vi "3_WF_Anomaly_Detection(Accuracy_Evaluation).vi"() -> ()   [LabVIEW 2020]
uses:
  <vilib>/Ngene/Deep Learning Toolkit/Toolkit/NN_Data/subVIs/Dataset/NN_Variant_to_DVR/2D/NN_Data_Variant_to_DVR(2D_SGL).vi
  <vilib>/Ngene/Deep Learning Toolkit/Toolkit/NN_Network/subVIs/NN_Predict/NN_Predict(In1D_Out1D).vi
  <vilib>/Ngene/Deep Learning Toolkit/Toolkit/NN_Data/subVIs/Get_Data_Vals/2D/NN_Data_Get_ValByRef(2D_SGL).vi
  <vilib>/Ngene/Deep Learning Toolkit/Toolkit/Deep_Learning_Toolkit_by_Ngene.lvlib
  <vilib>/Analysis/NI_AALPro.lvlib
panel:
  out "Error Rate":sgl
  in  "Labels":string[](array[string])=["Normal", "Abnormal"]
  in  "Optimal Threshold":sgl=0.2
  out "Anomaly Score Distribution":T1(graph)=[{"X Values"=array[700 elements], "Histogram: h(x)"=[0, 0, 0, 0, 0, 0, 0, 0, 0, 0, 0, 0, 0, 0, 0, 0, 0, 0, 0, 0, 0, 0, 0, 0, 0, 0, 0, 0, 0, 0, 0, 0, 0, 0, 0, 1, 0, 1, 2, 2, 7, 7, 7, 4, 17, 6, 12, 11, 9, 10, 15, 15, 11, 18, 18, 18, 13, 13, 16, 11, 14, 20, 11, 9, 16, 11, 16, 10, 11, 9, 8, 15, 6, 8, 4, 10, 3, 4, 1, 6, 3, 6, 3, 10, 6, 5, 3, 1, 5, 2, 1, 2, 1, 4, 2, 2, 1, 1, 0, 1, 0, 0, 1, 0, 0, 0, 1, 1, 0, 0, 0, 0, 0, 0, 0, 0, 1, 0, 0, 0, 0, 0, 0, 1, 0, 0, 0, 0, 0, 0, 0, 0, 0, 0, 0, 0, 0, 0, 0, 0, 0, 0, 0, 0, 0, 0, 0, 0, 0, 0, 0, 0, 0, 0, 0, 0, 0, 0, 0, 0, 0, 0, 0, 0, 0, 0, 0, 0, 0, 0, 0, 0, 0, 0, 0, 0, 0, 0, 0, 0, 0, 0, 0, 0, 0, 0, 0, 0, 0, 0, 0, 0, 0, 0, 0, 0, 0, 0, 0, 0, 0, 0, 0, 0, 0, 0, 0, 0, 0, 0, 0, 0, 0, 0, 0, 0, 0, 0, 0, 0, 0, 0, 0, 0, 0, 0, 0, 0, 0, 0, 0, 0, 0, 0, 0, 0, 0, 0, 0, 0, 0, 0, 0, 0, 0, 0, 0, 0, 0, 0, 0, 0, 0, 0, 0, 0, 0, 0, 0, 0, 0, 0, 0, 0, 0, 0, 0, 0, 0, 0, 0, 0, 0, 0, 0, 0, 0, 0, 0, 0, 0, 0, 0, 0, 0, 0, 0, 0, 0, 0, 0, 0, 0, 0, 0, 0, 0, 0, 0, 0, 0, 0, 0, 0, 0, 0, 0, 0, 0, 0, 0, 0, 0, 0, 0, 0, 0, 0, 0, 0, 0, 0, 0, 0, 0, 0, 0, 0, 0, 0, 0, 0, 0, 0, 0, 0, 0, 0, 0, 0, 0, 0, 0, 0, 0, 0, 0, 0, 0, 0, 0, 0, 0, 0, 0, 0, 0, 0, 0, 0, 0, 0, 0, 0, 0, 0, 0, 0, 0, 0, 0, 0, 0, 0, 0, 0, 0, 0, 0, 0, 0, 0, 0, 0, 0, 0, 0, 0, 0, 0, 0, 0, 0, 0, 0, 0, 0, 0, 0, 0, 0, 0, 0, 0, 0, 0, 0, 0, 0, 0, 0, 0, 0, 0, 0, 0, 0, 0, 0, 0, 0, 0, 0, 0, 0, 0, 0, 0, 0, 0, 0, 0, 0, 0, 0, 0, 0, 0, 0, 0, 0, 0, 0, 0, 0, 0, 0, 0, 0, 0, 0, 0, 0, 0, 0, 0, 0, 0, 0, 0, 0, 0, 0, 0, 0, 0, 0, 0, 0, 0, 0, 0, 0, 0, 0, 0, 0, 0, 0, 0, 0, 0, 0, 0, 0, 0, 0, 0, 0, 0, 0, 0, 0, 0, 0, 0, 0, 0, 0, 0, 0, 0, 0, 0, 0, 0, 0, 0, 0, 0, 0, 0, 0, 0, 0, 0, 0, 0, 0, 0, 0, 0, 0, 0, 0, 0, 0, 0, 0, 0, 0, 0, 0, 0, 0, 0, 0, 0, 0, 0, 0, 0, 0, 0, 0, 0, 0, 0, 0, 0, 0, 0, 0, 0, 0, 0, 0, 0, 0, 0, 0, 0, 0, 0, 0, 0, 0, 0, 0, 0, 0, 0, 0, 0, 0, 0, 0, 0, 0, 0, 0, 0, 0, 0, 0, 0, 0, 0, 0, 0, 0, 0, 0, 0, 0, 0, 0, 0, 0, 0, 0, 0, 0, 0, 0, 0, 0, 0, 0, 0, 0, 0, 0, 0, 0, 0, 0, 0, 0, 0, 0, 0, 0, 0, 0, 0, 0, 0, 0, 0, 0, 0, 0, 0, 0, 0, 0, 0, 0, 0, 0, 0, 0, 0, 0, 0, 0, 0, 0, 0, 0, 0, 0, 0, 0, 0, 0, 0, 0, 0, 0, 0, 0, 0, 0, 0, 0, 0, 0, 0, 0, 0, 0, 0, 0, 0, 0, 0, 0, 0, 0, 0, 0, 0, 0, 0, 0, 0, 0, 0, 0, 0, 0, 0, 0, 0, 0, 0, 0, 0]}, {"X Values"=array[700 elements], "Histogram: h(x)"=[0, 0, 0, 0, 0, 0, 0, 0, 0, 0, 0, 0, 0, 0, 0, 0, 0, 0, 0, 0, 0, 0, 0, 0, 0, 0, 0, 0, 0, 0, 0, 0, 0, 0, 0, 0, 0, 0, 0, 0, 0, 0, 0, 0, 0, 0, 0, 0, 0, 0, 0, 0, 0, 0, 0, 0, 0, 0, 0, 0, 0, 0, 0, 0, 0, 0, 0, 0, 0, 0, 0, 0, 0, 0, 0, 0, 0, 0, 0, 0, 0, 0, 0, 0, 0, 0, 0, 0, 0, 0, 0, 0, 0, 0, 0, 0, 0, 0, 0, 0, 0, 0, 0, 0, 0, 0, 0, 0, 0, 0, 0, 0, 0, 0, 0, 0, 0, 0, 0, 0, 0, 0, 0, 0, 0, 0, 0, 0, 0, 0, 0, 0, 0, 0, 0, 0, 0, 0, 0, 0, 0, 0, 0, 0, 0, 0, 0, 0, 0, 0, 0, 0, 0, 0, 0, 0, 0, 0, 0, 0, 0, 0, 0, 0, 0, 0, 0, 0, 0, 1, 0, 0, 0, 0, 0, 2, 0, 0, 0, 0, 0, 0, 0, 0, 1, 1, 2, 1, 2, 0, 2, 0, 1, 0, 0, 0, 1, 1, 1, 1, 2, 3, 2, 0, 1, 0, 2, 3, 1, 2, 0, 4, 4, 1, 0, 1, 1, 0, 0, 0, 1, 0, 4, 3, 2, 5, 2, 2, 1, 1, 2, 1, 4, 3, 2, 1, 2, 5, 0, 4, 1, 1, 3, 2, 2, 2, 1, 2, 6, 2, 1, 0, 0, 2, 1, 3, 2, 3, 6, 1, 4, 5, 0, 1, 1, 4, 3, 2, 5, 2, 2, 0, 1, 0, 2, 0, 2, 4, 0, 2, 0, 2, 0, 4, 1, 0, 1, 1, 0, 1, 1, 3, 3, 1, 0, 0, 3, 1, 1, 0, 1, 1, 1, 4, 2, 2, 3, 0, 1, 1, 3, 1, 1, 0, 0, 0, 2, 0, 1, 3, 1, 0, 1, 1, 1, 0, 1, 0, 1, 1, 0, 0, 0, 0, 1, 2, 1, 0, 1, 0, 0, 0, 0, 0, 0, 0, 3, 2, 0, 0, 0, 1, 0, 0, 0, 2, 0, 0, 1, 0, 1, 2, 2, 4, 2, 1, 2, 3, 1, 1, 3, 0, 1, 3, 1, 2, 0, 1, 0, 1, 0, 2, 1, 1, 1, 2, 1, 0, 2, 0, 1, 1, 2, 4, 4, 2, 2, 0, 1, 2, 1, 1, 1, 1, 1, 1, 1, 1, 2, 1, 1, 1, 1, 5, 3, 1, 1, 1, 4, 2, 3, 1, 0, 0, 1, 0, 0, 0, 1, 5, 2, 1, 2, 1, 1, 3, 0, 3, 2, 2, 0, 1, 1, 2, 1, 0, 2, 1, 2, 0, 1, 0, 1, 2, 0, 1, 0, 0, 2, 0, 0, 0, 2, 1, 2, 1, 2, 1, 1, 1, 1, 0, 1, 1, 0, 1, 1, 0, 1, 1, 0, 0, 0, 0, 0, 1, 0, 0, 0, 1, 0, 0, 0, 0, 0, 0, 0, 0, 0, 0, 0, 1, 0, 0, 0, 0, 0, 0, 0, 0, 0, 1, 0, 0, 0, 0, 0, 0, 0, 0, 0, 0, 0, 0, 0, 0, 0, 0, 0, 0, 0, 0, 0, 0, 0, 0, 1, 0, 0, 0, 0, 0, 0, 0, 0, 0, 0, 0, 0, 0, 0, 0, 0, 0, 0, 0, 0, 0, 0, 0, 0, 0, 0, 0, 0, 0, 0, 1, 1, 0, 0, 0, 0, 0, 1, 1, 1, 0, 0, 0, 0, 0, 0, 1, 0, 0, 3, 0, 1, 0, 0, 0, 0, 2, 2, 0, 4, 0, 3, 3, 1, 0, 1, 4, 4, 1, 3, 1, 0, 2, 1, 2, 1, 3, 1, 1, 0, 1, 0, 5, 2, 4, 4, 2, 1, 1, 0, 1, 1, 2, 1, 2, 3, 2, 1, 1, 1, 3, 0, 0, 1, 4, 1, 0, 0, 2, 0, 0, 2, 0, 0, 0, 0, 0, 0, 1, 0, 0, 1, 0, 0, 0, 0, 0, 0, 0, 0, 0, 0, 0, 0, 0, 0, 0, 0, 0, 0, 0, 0, 0, 0, 0, 0, 0, 0, 0, 0, 0, 0, 0, 0, 0, 0, 0, 0, 0, 0, 0, 0, 0]}]
  in  "Test (Normal Samples) Dataset Folder path":path=path "D:/working/Anomaly Detection/Test/Normal"
  out "Confusion Matrix (Table)":string[][](table)=[["500", "0", "1.0000"], ["0", "500", "1.0000"], ["1.0000", "1.0000", ""]]
  in  "Test (Abnormal Samples) Dataset Folder path":path=path "D:/working/Anomaly Detection/Test/Abnormal"
  in  "Weights File Path":path=path "D:/Ngene/GitHub/deepltk_examples/2_Waveform_Processing/24_Waveform_Anomaly_Detection/working/Anomaly_Detection/Anomaly_Detection_weights_25_06_11__13_26_24.bin"
  in  "CFG file path":path=path "D:/Ngene/GitHub/deepltk_examples/2_Waveform_Processing/24_Waveform_Anomaly_Detection/working/Anomaly_Detection/Anomaly_Detection_net_cfg_25_06_11__13_26_24.cfg"
  # "Overview: This VI is designed to calculate the optimal anomaly threshold on the generated synthetic dataset.\nRequirements: Deep Learning Toolkit for LabVIEW - https://www.ngene.co/deep-learning-toolkit-for-labview\nInstructions:\n1. Provide \"Network Configuration File Path\" and \"Weight File Path\" generated from \"1_WF_Anomaly_Detection(Training).vi\".\n2. Provide Train and Test dataset paths.\n3. Run the VI.\n4.Observe the Range of optimal threshold values.\n5. Choose a value from the range of optimal threshold calculated after the VI stops, and use it as a anomaly detetcion threshold in \"3_WF_Anomaly_Detection(Threshold_Evaluation).vi\" \n6. Open \"3_WF_Anomaly_Detection(Inference).vi\"  to deploy the trained network for inference on manually generated samples."
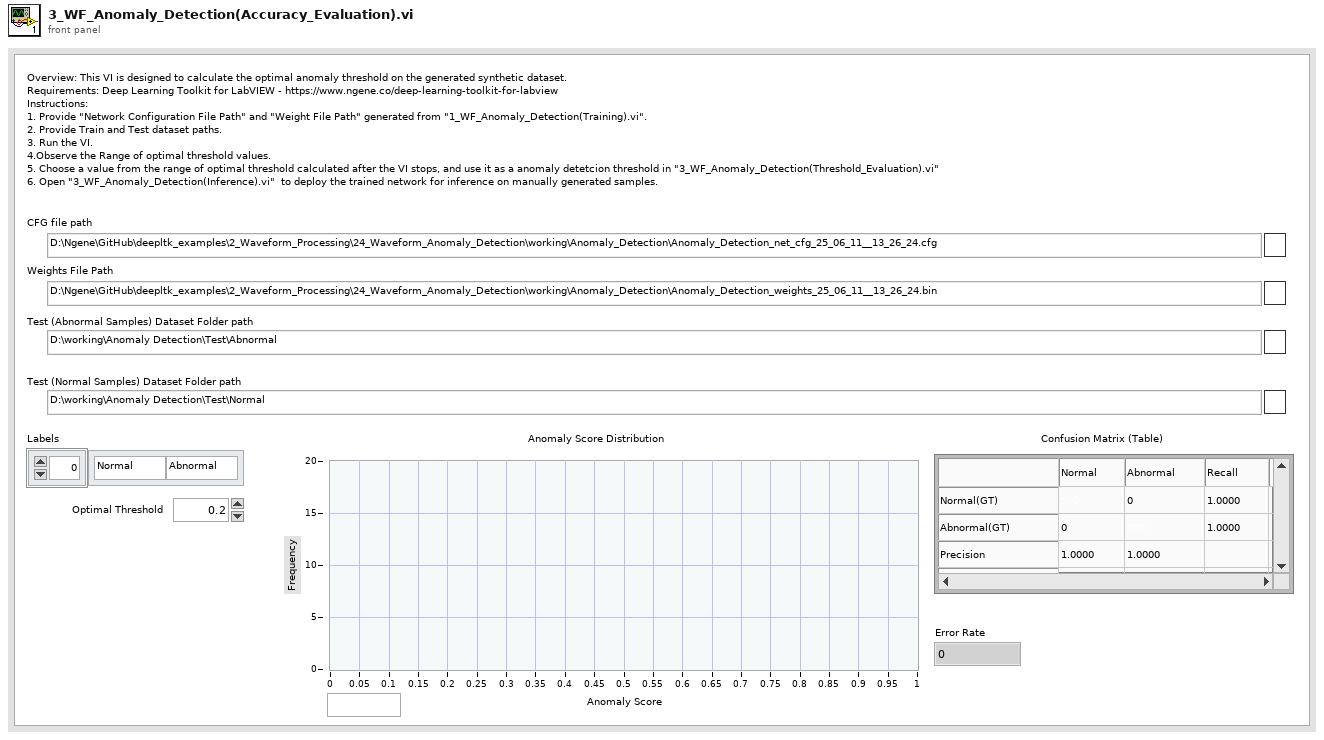
[diagram p1: front panel]
types:
  T1 = cluster{"X Values":dbl[], "Histogram: h(x)":i32[]}[]
  T2 = typedef "Deep_Learning_Toolkit_by_Ngene.lvlib/NN_Config_Params.ctl" = cluster{"Name":string, "mBatch":i32, "NN_Train_Params":T3, "LR_Decay_Policy":T6, "Labels":string[], "Loss":T8}
  T3 = typedef "Deep_Learning_Toolkit_by_Ngene.lvlib/NN_Train_Params.ctl" = cluster{"Optimizer":T4, "Beta_1":sgl, "Beta_2":sgl, "Weight Decay(L1)":sgl, "Weight Decay(L2)":sgl, "Data_Sampling":T5}
  T4 = typedef "Deep_Learning_Toolkit_by_Ngene.lvlib/NN_Train_Optimizer.ctl" = enum16{"SGD", "Adam", "Adagrad", "Adadelta", "RMSProp", "Nesterov"}
  T5 = typedef "Deep_Learning_Toolkit_by_Ngene.lvlib/NN_Train_Data_Sampling.ctl" = enum16{"Random", "Sequential"}
  T6 = typedef "Deep_Learning_Toolkit_by_Ngene.lvlib/NN_LR_Policy_Cfg.ctl" = cluster{"Policy_Type":T7, "LR0":dbl, "k":sgl, "WarmUp_Policy":enum16{"Step", "Ramp"}, "WarmUp_Iter":i32, "WarmUp_Ratio":sgl}
  T7 = typedef "Deep_Learning_Toolkit_by_Ngene.lvlib/NN_LR_Policy_Type.ctl" = enum16{"Manual", "Step", "Exp", "1/t"}
  T8 = typedef "Deep_Learning_Toolkit_by_Ngene.lvlib/NN_Loss_Config_Params.ctl" = cluster{"Loss_Type":T9, "Loss_Conf_Params":variant}
  T9 = typedef "Deep_Learning_Toolkit_by_Ngene.lvlib/NN_Loss_Type.ctl" = enum16{"None", "MSE", "CrossEntropy", "YOLO_v2", "YOLO_v4"}
  T10 = typedef "Deep_Learning_Toolkit_by_Ngene.lvlib/NN_Layer_Config_Params.ctl" = cluster{"Layer_Type":T11, "Layer_Conf_Params":variant, "Input Layers":string[]}
  T11 = typedef "Deep_Learning_Toolkit_by_Ngene.lvlib/NN_Layer_Type.ctl" = enum16{"Input1D", "Input3D", "Conv1D", "Conv2D", "Conv2D_Adv", "MaxPool", "AvgPool", "UpSample", "DropOut3D", "ShortCut", "Concat", "SoftMax3D", "FC", "DropOut", "Softmax", "Flatten", "YOLO_v2", "YOLO_v4", "Activation", "BatchNormalization", "Unsupported"}
  T12 = typedef "Deep_Learning_Toolkit_by_Ngene.lvlib/NN.ctl" = cluster{"Name":string, "No of Layers":i32, "mBatch":i32, "Layers":T13[], "Dimty":T14, "Dims_In":T15, "Dims_Out":T15, "Working_Dir":path, "Train?":bool, "Train_Params":T3, "LR_Update_Policy":T6, "Session Data":T16, "Ground_truth":T17, "NNg_hdls":T18, "NN_Device":T19, "GPU Id":i32, "Labels":string[], "Receptive Field":T20[], "Loss_Type":T9, "Loss_Cfg_Prms":variant, "NNG_WS":T21}
  T13 = typedef "Deep_Learning_Toolkit_by_Ngene.lvlib/NN_Layer_ref.ctl" = refnum<data-value>
  T14 = typedef "Deep_Learning_Toolkit_by_Ngene.lvlib/NN_In_Out_Dim-ty.ctl" = enum8{"In1D_Out1D", "In3D_Out1D", "In3D_Out3D", "In3D_OutBBox"}
  T15 = typedef "Deep_Learning_Toolkit_by_Ngene.lvlib/NN_Dims(C,H,W).ctl" = cluster{"C":i32, "H":i32, "W":i32}
  T16 = typedef "Deep_Learning_Toolkit_by_Ngene.lvlib/NN_Train_Session_Data.ctl" = cluster{"Epochs":sgl, "Tot_Iter":i32, "LR":sgl, "LR_iter":i32}
  T17 = typedef "Deep_Learning_Toolkit_by_Ngene.lvlib/NN_Ground_truth.ctl" = cluster{"Y":variant}
  T18 = typedef "Deep_Learning_Toolkit_by_Ngene.lvlib/nng_cuda_handles.ctl" = cluster{"cudnn":u64, "cublas":u64, "stream":u64, "curand":u64}
  T19 = typedef "Deep_Learning_Toolkit_by_Ngene.lvlib/NN_Device.ctl" = enum16{"CPU", "GPU"}
  T20 = typedef "Deep_Learning_Toolkit_by_Ngene.lvlib/NN_Dims(V,H).ctl" = cluster{"V":i32, "H":i32}
  T21 = typedef "Deep_Learning_Toolkit_by_Ngene.lvlib/NNG_WS.ctl" = cluster{"NNG_WS_Mem":T22, "Max_WS_Size":i64}
  T22 = typedef "Deep_Learning_Toolkit_by_Ngene.lvlib/NNg_WS_Mem_DVR.ctl" = refnum<data-value>
  T23 = typedef "Deep_Learning_Toolkit_by_Ngene.lvlib/NN_DataSet(In1D_Out1D).ctl" = cluster{"Inputs Ref.":variant, "Outputs Ref.":T24, "Dims_In":i32, "Dataset_Size":i32, "Dims_Out":i32, "Labels":string[], "File Paths":path[]}
  T24 = typedef "Deep_Learning_Toolkit_by_Ngene.lvlib/NN_Data_ref(2D_SGL).ctl" = refnum<data-value>
  T25 = cluster{"X Values":dbl[], "Histogram: h(x)":i32[]}
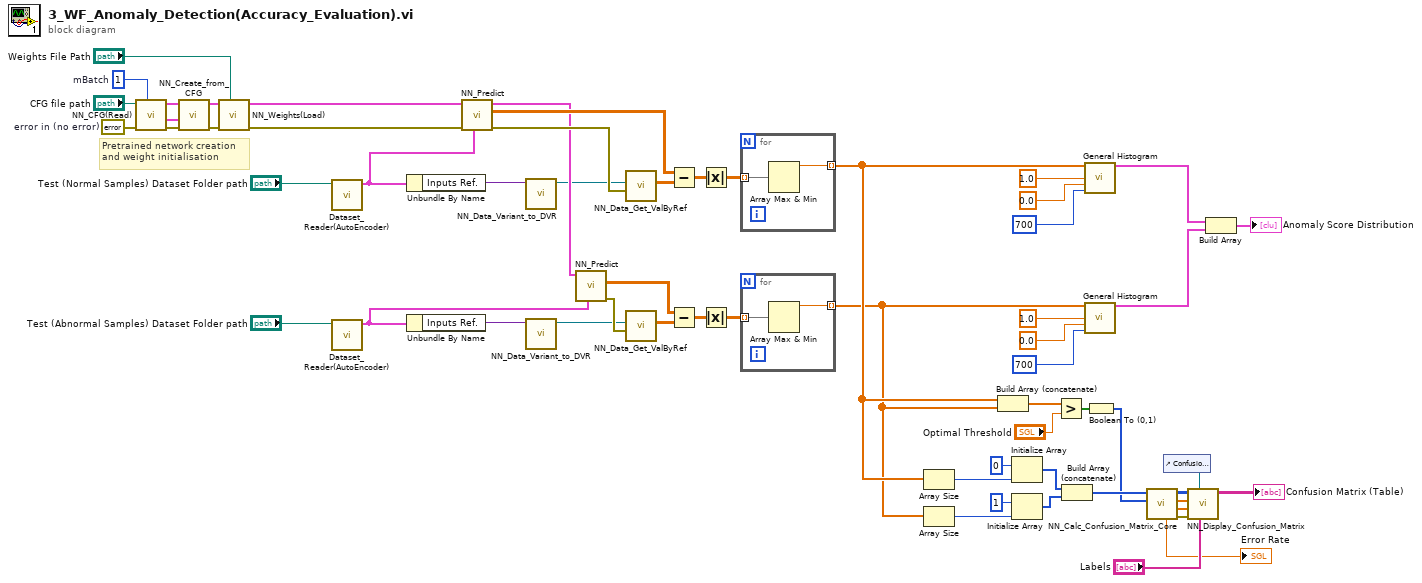
[diagram p0: block diagram]
diagram:
  w54 = 1  # mBatch
  w59 = errorcluster {"status"=FALSE, "code"=0, "source"=""}  # error in (no error)
  # "Pretrained network creation\nand weight initialisation"
  n1 = call <vilib>:"NN_CFG(Read).vi"("mBatch"=w54, "error in (no error)"=w59, "CFG file path"="CFG file path") -> ("error out"=w57:errorcluster, "Net_Cfg"=w58:T2, "Layer_Cfg"=w56:T10[])  [unwired: 6 in]
  n2 = call <vilib>:"NN_Create_from_CFG.vi"("error in (no error)"=w57, "Net_Cfg"=w58, "Layer_Cfg"=w56) -> ("error out"=w60:errorcluster, "NN out"=w55:T12)  [unwired: 7 in]
  n3 = call <vilib>:"NN_Weights(Load).vi"("Weight File Path"="Weights File Path", "error in (no error)"=w60, "NN in"=w55) -> ("error out"=w43:errorcluster, "NN out"=w44:T12)  [unwired: 7 in]
  n4 = call "Dataset_Reader(AutoEncoder).vi"("Train dataset path"="Test (Normal Samples) Dataset Folder path") -> ("Dataset"=w34:T23)  [unwired: 9 in, 1 out]
  n5 = call "Dataset_Reader(AutoEncoder).vi"("Train dataset path"="Test (Abnormal Samples) Dataset Folder path") -> ("Dataset"=w37:T23)  [unwired: 9 in, 1 out]
  n6 = Unbundle By Name(w34) -> ("Inputs Ref."=w41:variant)
  n7 = Unbundle By Name(w37) -> ("Inputs Ref."=w36:variant)
  n8 = call-poly <vilib>:"NN_Predict.vi"("Dataset"=w34, "error in (no error)"=w43, "NN in"=w44) -> ("error out"=w51:errorcluster, "Predictions"=w40:sgl[][], "NN out"=w38:T12)  [unwired: 6 in]
  n9 = call-poly <vilib>:"NN_Data_Variant_to_DVR.vi"("Inputs Ref."=w41) -> ("DVR(2D_SGL)"=w2:T24)  [unwired: 9 in, 1 out]
  n10 = call-poly <vilib>:"NN_Data_Variant_to_DVR.vi"("Inputs Ref."=w36) -> ("DVR(2D_SGL)"=w1:T24)  [unwired: 9 in, 1 out]
  n11 = call-poly <vilib>:"NN_Predict.vi"("Dataset"=w37, "NN in"=w38) -> ("error out"=w39:errorcluster, "Predictions"=w28:sgl[][])  [unwired: 7 in, 1 out]
  n12 = call-poly <vilib>:"NN_Data_Get_ValByRef.vi"("error in (no error)"=w51, "DVR(2D_SGL)"=w2) -> ("Value(2D_SGL)"=w50:sgl[][])  [unwired: 6 in, 1 out]
  n13 = call-poly <vilib>:"NN_Data_Get_ValByRef.vi"("error in (no error)"=w39, "DVR(2D_SGL)"=w1) -> ("Value(2D_SGL)"=w29:sgl[][])  [unwired: 6 in, 1 out]
  n14 = Subtract(x=w40, y=w50) -> (x-y=w49:sgl[][])
  n15 = Subtract(x=w28, y=w29) -> (x-y=w30:sgl[][])
  n16 = Absolute Value(x=w49) -> (abs(x)=w48:sgl[][])
  n17 = Absolute Value(x=w30) -> (abs(x)=w31:sgl[][])
  n18 = for {
    tunnel: w48 -> [w62] mode=indexing
    tunnel: [w61] -> w8 mode=indexing
    n19 = Array Max & Min(array=w62) -> (max value=w61:sgl)  [unwired: 3 out]
  }
  n20 = for {
    tunnel: w31 -> [w64] mode=indexing
    tunnel: [w63] -> w7 mode=indexing
    n21 = Array Max & Min(array=w64) -> (max value=w63:sgl)  [unwired: 3 out]
  }
  n22 = Array Size(array=w8) -> (size(s)=w17:i32)
  n23 = Array Size(array=w7) -> (size(s)=w12:i32)
  n24 = Build Array (concatenate)(w8, w7) -> (w9:sgl[])
  n25 = Initialize Array(0 ("element"), w17) -> (w15:i32[])
  n26 = Initialize Array(1 ("element"), w12) -> (w13:i32[])
  n27 = Greater?(x=w9, y="Optimal Threshold") -> (0:w6:bool[])
  n28 = Build Array (concatenate)(w15, w13) -> (w11:i32[])
  n29 = call <vilib>:"General Histogram.vi"("X"=w8, "max"=1.0, "min"=0.0, "# bins"=700) -> ("Histogram Graph"=w26:T25)  [unwired: 7 in, 4 out]
  n30 = call <vilib>:"General Histogram.vi"("X"=w7, "max"=1.0, "min"=0.0, "# bins"=700) -> ("Histogram Graph"=w25:T25)  [unwired: 7 in, 4 out]
  n31 = Boolean To (0,1)(Boolean=w6) -> (0, 1=w5:i16[])
  n32 = call <vilib>:"NN_Calc_Confusion_Matrix_Core.vi"("Predictions"=w5, "Ground_Truths"=w11) -> ("Error Out"=w20:errorcluster, "Recall"=w21:sgl[], "Precision"=w22:sgl[], "Confusion Matrix"=w23:i32[][], "Error Rate"=→"Error Rate":sgl)  [unwired: 5 in]
  n33 = control-ref of="Confusion Matrix (Table)"() -> (w19:refnum<vi>)
  n34 = call <vilib>:"NN_Display_Confusion_Matrix.vi"("Labels"="Labels", "Confusion Matrix (Table) ref"=w19, "error in (no error)"=w20, "Recall"=w21, "Precision"=w22, "Confusion Matrix"=w23) -> ("Confusion Matrix (Table)"=→"Confusion Matrix (Table)":string[][])  [unwired: 4 in, 1 out]
  n35 = Build Array(w26, w25) -> (→"Anomaly Score Distribution":T1)
